vi "Find Mode.vi"(8 "move count":i32, 9 "Column":i32, 10 "Row":i32, 11 "private data in":T4) -> (0 "distance":dbl, 1 "nearest wall":T3, 2 "mode":T2, 3 "private data out":T4, 4 "even?":bool, 6 "wall state":T1)   [LabVIEW 2020, in "Great Wall.lvclass"]
uses:
  Great Wall.lvclass
  Private Data.ctl
  Wall State.ctl
  Wall State Enum.ctl
  Type Defs/Direction Enum.ctl
  Square Mode.ctl
  SubVIs/Read-Only Globals.vi
  SubVIs/Globals (private).vi
  DS Square Library/DS Square.lvlib
  Square/Square.lvclass
  Type Defs/SB Type Defs.lvlib
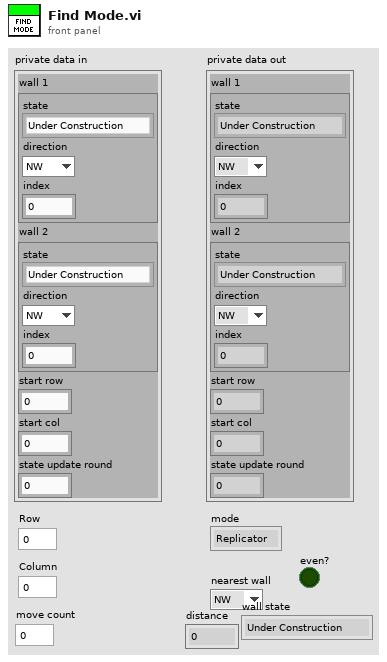
[diagram p1: front panel]
types:
  T1 = typedef "Great Wall.lvclass/Wall State Enum.ctl" = enum16{"Under Construction", "Hold", "Advance 1", "Advance 2", "Retreat"}
  T2 = typedef "Great Wall.lvclass/Square Mode.ctl" = enum16{"Replicator", "Guard", "Wall"}
  T3 = typedef "SB Type Defs.lvlib/Direction Enum.ctl" = enum16{"NW", "N", "NE", "E", "SE", "S", "SW", "W"}
  T4 = typedef "Great Wall.lvclass/Private Data.ctl" = cluster{"wall 1":T5, "wall 2":T5, "start row":i32, "start col":i32, "state update round":i32}
  T5 = typedef "Great Wall.lvclass/Wall State.ctl" = cluster{"state":T1, "direction":T3, "index":i32}
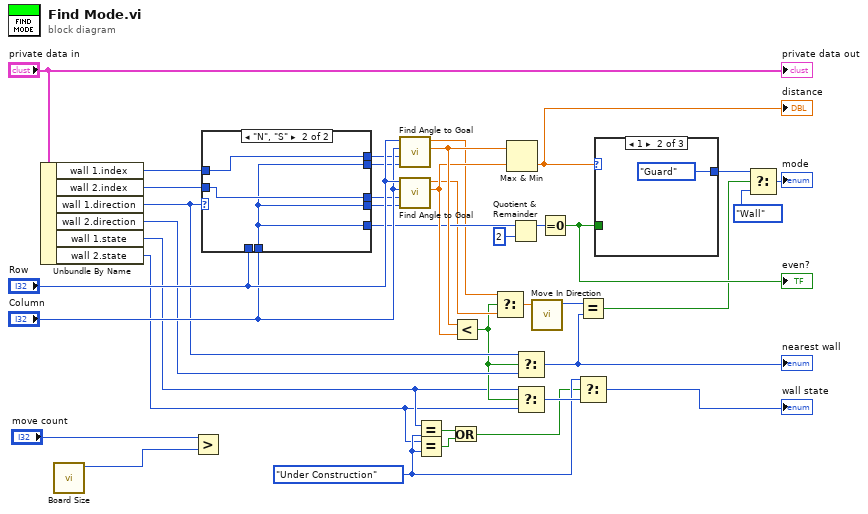
[diagram p0: block diagram]
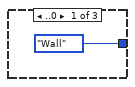
[diagram p2: hidden frame]
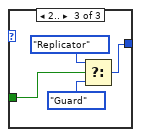
[diagram p3: hidden frame]
diagram:
  w6 = Wall_State_Enum."Under Construction" ("f")
  n1 = Unbundle By Name("private data in") -> ("wall 1.index"=w37:i32, "wall 2.index"=w38:i32, "wall 1.direction"=w28:T3, "wall 2.direction"=w29:T3, "wall 1.state"=w5:T1, "wall 2.state"=w4:T1)
  n2 = call "Board Size.vi"() -> ("Board Size"=w19:i32)  [unwired: 11 in]
  n3 = Greater?(x="move count", y=w19) -> ()  [unwired: 1 out]
  n4 = case shown="\"N\", \"S\"" w28 {
    tunnel: "Row" -> [w39 _]
    tunnel: "Column" -> [_ w42]
    tunnel: w38 -> [w41 w43]
    tunnel: w37 -> [w40 w44]
    tunnel: [w39 w44] -> w34
    tunnel: [w39 w43] -> w33
    tunnel: [w41 w42] -> w32
    tunnel: [w40 w42] -> w31
    tunnel: [w39 w42] -> w24
    frame "E", "W", Default {
    }
    frame "N", "S" {
    }
  }
  n5 = call "Find Angle to Goal.vi"("Goal Column"=w31, "Goal Row"=w34, "Column"="Column", "Row"="Row") -> ("distance"=w27:dbl, "angle (deg)"=w17:dbl)  [unwired: 4 in, 2 out]
  n6 = call "Find Angle to Goal.vi"("Goal Column"=w32, "Goal Row"=w33, "Column"="Column", "Row"="Row") -> ("distance"=w26:dbl, "angle (deg)"=w18:dbl)  [unwired: 4 in, 2 out]
  n7 = Equal?(x=w5, y=w6) -> (x = y?=w3:bool)
  n8 = Equal?(x=w4, y=w6) -> (x = y?=w2:bool)
  n9 = Or(x=w3, y=w2) -> (x .or. y?=w1:bool)
  n10 = Less?(x=w27, y=w26) -> (x < y?=w9:bool)
  n11 = Select(t=w17, s=w9, f=w18) -> (s? t:f=w16:dbl)
  n12 = Max & Min(x=w27, y=w26) -> (min(x,y)=w25:dbl)  [unwired: 1 out]
  "distance" <- w25
  n13 = Quotient & Remainder(x=w24, y=2) -> (x-y*floor(x/y)=w22:i32)  [unwired: 1 out]
  n14 = Select(t=w28, s=w9, f=w29) -> (s? t:f=w10:T3)
  "nearest wall" <- w10
  n15 = Select(t=w5, s=w9, f=w4) -> (s? t:f=w8:T1)
  n16 = call "Move In Direction.vi"("goal angle (deg)"=w16) -> ("best direction"=w15:T3)  [unwired: 9 in, 1 out]
  n17 = Equal To 0?(x=w22) -> (x = 0?=w21:bool)
  "even?" <- w21
  n18 = Equal?(x=w15, y=w10) -> (x = y?=w14:bool)
  n19 = Select(t=w6, s=w1, f=w8) -> (s? t:f=→"wall state":T1)
  n20 = case shown="1" w25 {
    tunnel: [Square_Mode."Wall" ("mode") Square_Mode."Guard" ("mode") w47] -> w13
    tunnel: w21 -> [_ _ w50]
    frame ..0 {
    }
    frame 1 {
    }
    frame 2.. {
      n21 = Select(t=Square_Mode."Replicator" ("mode"), s=w50, f=Square_Mode."Guard" ("mode")) -> (s? t:f=w47:T2)
    }
  }
  n22 = Select(t=w13, s=w14, f=Square_Mode."Wall" ("mode")) -> (s? t:f=→"mode":T2)
  "private data out" <- "private data in"
